vi "Write Reboot.vi"(8 "error in (no error)":errorcluster, 10 "Reboot":bool, 11 "Cobra GUI in":refnum<class "Cobra GUI.lvclass">) -> (0 "error out":errorcluster, 3 "Cobra GUI out":refnum<class "Cobra GUI.lvclass">)   [LabVIEW 2019]
uses:
  Cobra GUI.lvclass
  C:/Program Files (x86)/National Instruments/LabVIEW 2019/vi.lib/MGI/Panel Manager/Panel Actor/Panel Actor/Panel Actor.lvclass
  C:/Program Files (x86)/National Instruments/LabVIEW 2019/vi.lib/MGI/Monitored Actor/Monitored Actor/Monitored Actor/Monitored Actor.lvclass
  C:/Program Files (x86)/National Instruments/LabVIEW 2019/vi.lib/ActorFramework/Actor/Actor.lvclass
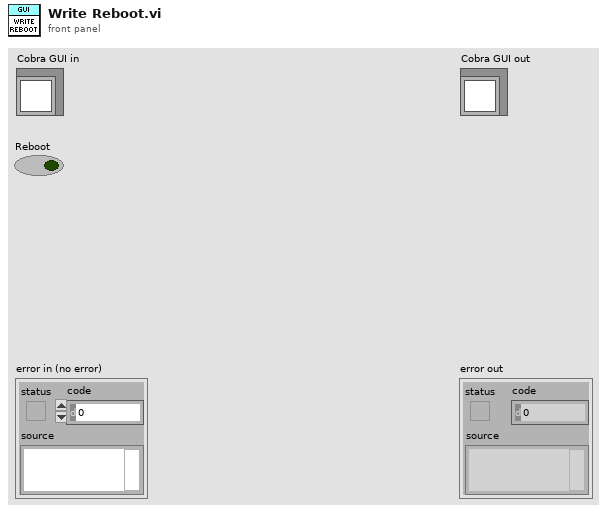
[diagram p1: front panel]
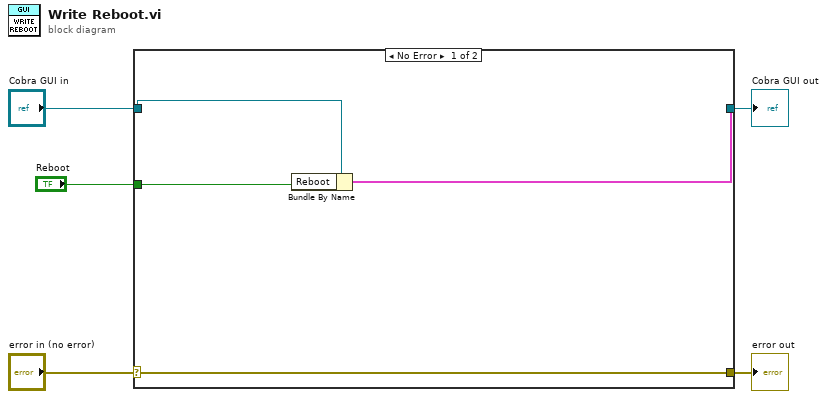
[diagram p0: block diagram]
diagram:
  n1 = case shown="No Error" "error in (no error)" {
    selector: "error in (no error)" -> [w9 w11]
    tunnel: [w9 w11] -> w4
    tunnel: [w7 w10] -> w2
    tunnel: "Cobra GUI in" -> [w8 w10]
    tunnel: "Reboot" -> [w6 _]
    frame No Error {
      n2 = Bundle By Name(cluster=w8, "Reboot"=w6) -> (w7:cluster{})
    }
    frame Error {
    }
  }
  "error out" <- w4
  "Cobra GUI out" <- w2
